vi "List My Dependencies Name.vi"(8 "error in (no error)":errorcluster, 9 "Fully Qualified Name? (F)":bool, 11 "SMO.E in":refnum<class "SMO.E.lvclass">) -> (0 "error out":errorcluster, 2 "Names":string[](array[string]), 3 "SMO.E out":refnum<class "SMO.E.lvclass">)   [LabVIEW 2013, in "SMO.E.lvclass"]
uses:
  SMO.E.lvclass
  src/SMO/SMO.lvclass
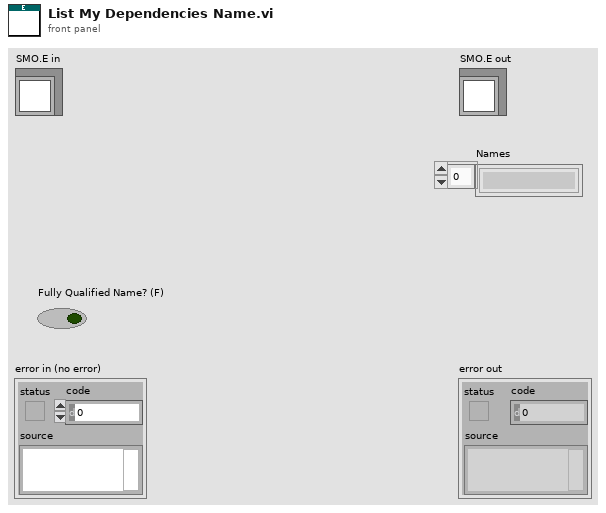
[diagram p1: front panel]
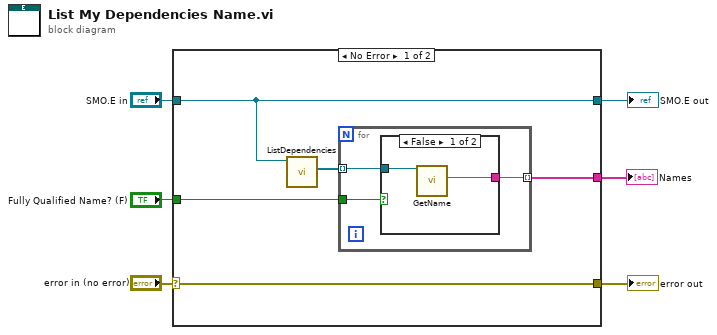
[diagram p0: block diagram]
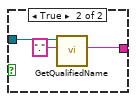
[diagram p2: hidden frame]
diagram:
  n1 = case shown="No Error" "error in (no error)" {
    selector: "error in (no error)" -> [w11 w21]
    tunnel: [w11 w21] -> w5
    tunnel: [w10 w20] -> w3
    tunnel: "SMO.E in" -> [w10 w20]
    tunnel: [w8 _] -> w2
    tunnel: "Fully Qualified Name? (F)" -> [w7 _]
    frame No Error {
      n2 = call "ListDependencies.vi"("SMO in"=w10) -> ("[Dependencies]"=w9:refnum<class "SMO.lvclass">[])  [unwired: 7 in, 3 out]
      n3 = for {
        tunnel: w9 -> [w14] mode=indexing
        tunnel: [w13] -> w8 mode=indexing
        tunnel: w7 -> [w12]
        n4 = case shown="False" w12 {
          tunnel: w14 -> [w16 w18]
          tunnel: [w15 w17] -> w13
          frame False {
            n5 = call "GetName.vi"("SMO"=w16) -> ("Name"=w15:string)  [unwired: 7 in, 3 out]
          }
          frame True {
            n6 = call "GetQualifiedName.vi"("separator (dot)"=".", "SMO"=w18) -> ("Qualified Name"=w17:string)  [unwired: 7 in, 2 out]
          }
        }
      }
    }
    frame Error {
    }
  }
  "error out" <- w5
  "SMO.E out" <- w3
  "Names" <- w2
